vi "NF WF1973_74 TOFF Ubas.vi"(6 "Read(F)":bool, 7 "Width(0)":dbl min=0.0 max=100.0 step=0.01 format="%.2f", 8 "error in (no error)":errorcluster caption="Error IN", 9 "Set Width(Input)":u16(ring) items=["Input", "Minimum", "Maximum"], 10 "Ch(Ch1)":bool, 11 "VISAsession":refnum<visa-resource-name>) -> (0 "error out":errorcluster caption="Error OUT", 2 "Query Width":dbl=999.0 format="%.2f", 3 "CopyVISAsession":refnum<visa-resource-name>)   [LabVIEW 2010]
panel:
  # "Choose\nInput"
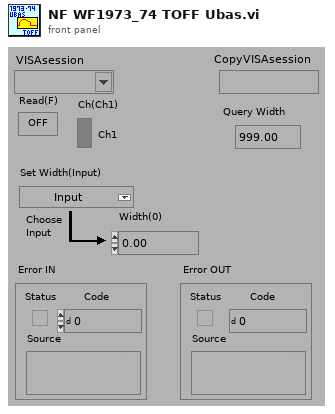
[diagram p1: front panel]
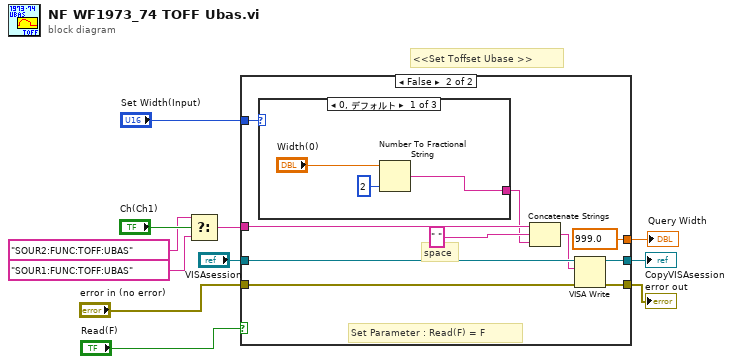
[diagram p0: block diagram]
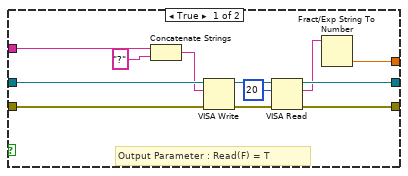
[diagram p2: hidden frame]
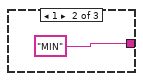
[diagram p3: hidden frame]
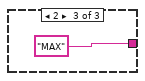
[diagram p4: hidden frame]
diagram:
  # "<<Set Toffset Ubase >>"
  n1 = Select(t="SOUR2:FUNC:TOFF:UBAS" ("文字列"), s="Ch(Ch1)", f="SOUR1:FUNC:TOFF:UBAS" ("文字列")) -> (s? t:f=w4:string)
  n2 = case shown="FALSE" "Read(F)" {
    tunnel: "VISAsession" -> [w23 w33]
    tunnel: [w20 w31] -> w10
    tunnel: [w19 w32] -> w9
    tunnel: "error in (no error)" -> [w18 w27]
    tunnel: w4 -> [w16 w28]
    tunnel: [w12 999.0] -> w6
    tunnel: "Set Width(Input)" -> [_ w26]
    frame True {
      # "Output Parameter : Read(F) = T"
      n3 = Concatenate Strings(w16, "?" ("形式文字列")) -> (w14:string)
      n4 = VISA Write(VISA resource name=w23, write buffer=w14, error in (no error)=w18) -> (VISA resource name out=w21:refnum<visa-resource-name>, error out=w22:errorcluster)  [unwired: 1 out]
      n5 = VISA Read(VISA resource name=w21, byte count=u32 20 ("バイトカウント（0）"), error in (no error)=w22) -> (VISA resource name out=w20:refnum<visa-resource-name>, read buffer=w13:string, error out=w19:errorcluster)  [unwired: 1 out]
      n6 = Fract/Exp String To Number(string=w13) -> (number=w12:dbl)  [unwired: 3 in, 1 out]
    }
    frame False {
      # "space"
      # "Set Parameter : Read(F) = F"
      n7 = case shown="0, デフォルト" w26 {
        tunnel: [w34 "MIN" ("文字列") "MAX" ("文字列")] -> w25
        frame 0, Default {
          n8 = Number To Fractional String(number="Width(0)", precision (6)=i16 2 ("精度 (6)")) -> (F-format string=w34:string)  [unwired: 2 in]
        }
        frame 1 {
        }
        frame 2 {
        }
      }
      n9 = Concatenate Strings(w28, " ", w25) -> (w30:string)
      n10 = VISA Write(VISA resource name=w33, write buffer=w30, error in (no error)=w27) -> (VISA resource name out=w31:refnum<visa-resource-name>, error out=w32:errorcluster)  [unwired: 1 out]
    }
  }
  "error out" <- w9
  "CopyVISAsession" <- w10
  "Query Width" <- w6
